vi "GetXML.vi"(0 "Node ROS":T2={"topic port"=0, "Node"="", "topic"="", "type"="", "node port"=0, "error "={"status"=FALSE, "code"=0, "source"=""}, "Direction"=enum."Node", "APIs"=[], "Update (ms)"=1, "write queue"=1}, 1 "Subscribers in":T1(array[cluster])) -> (2 "error IO":errorcluster, 3 "reply":string, 4 "Subscribers Out":T1(array[cluster]))   [LabVIEW 2012]
uses:
  ROSLog.ctl
  _ROSDefinition.vi
  MessageBuilding/std_msgs/subs/i16Scalar.vi
  MessageBuilding/std_msgs/subs/stringScalar.vi
  SubVIs/_ROSDirection.ctl
  SubVIs/_ROSControl.ctl
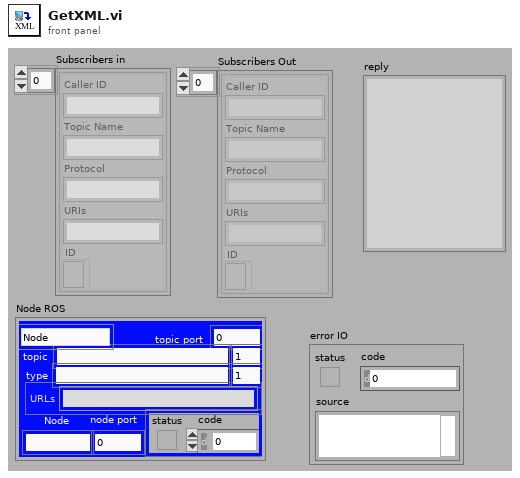
[diagram p1: front panel]
types:
  T1 = cluster{"Caller ID":string, "Topic Name":string, "Protocol":string, "URIs":string, "ID":refnum<k5>}[]
  T2 = typedef "_ROSControl.ctl" = cluster{"topic port":u16, "Node":string, "topic":string, "type":string, "node port":u32, "error ":errorcluster, "Direction":T3, "APIs":string[], "Update (ms)":u16, "write queue":u16}
  T3 = typedef "_ROSDirection.ctl" = enum16{"Node", "Publisher", "Subscriber", "Service Client"}
  T4 = typedef "ROSLog.ctl" = cluster{"Sent":string, "Reply":string, "MethodName":string, "success":bool, "Dir1":string, "Dir2":string, "Time Stamp":string}
  T5 = enum16{"Add Server", "Clear Server", "Clear All", "Get Info", "GetPanelInfo"}
  T6 = cluster{"Caller ID":string, "Topic Name":string, "Protocol":string, "URIs":string, "ID":refnum<k5>}
  T7 = typedef "requestTopic.ctl" = cluster{"New Subscriber":cluster{"Caller ID":string, "Topic Name":string, "Protocol":string, "URIs":string, "ID":refnum<k5>}, "ROS of Server":T2, "new port":u16}
  T8 = typedef "MyState.ctl" = enum16{"No Connection", "Registered", "Connected", "Close"}
  T9 = typedef "ServoInfo.ctl" = cluster{"vi name":string, "VI Refnum":refnum<vi>, "queue":refnum<queue>, "ROS":T2, "notifier":refnum<notifier>}
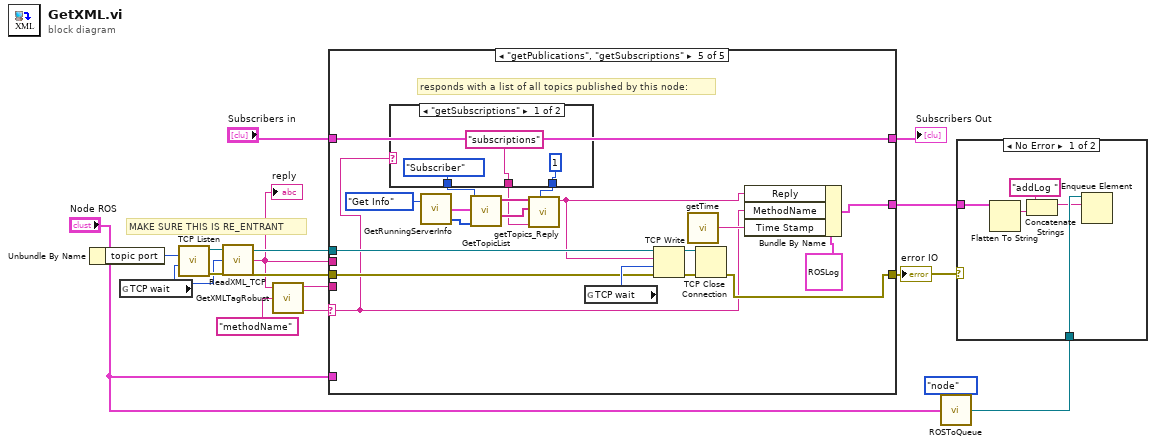
[diagram p0: block diagram]
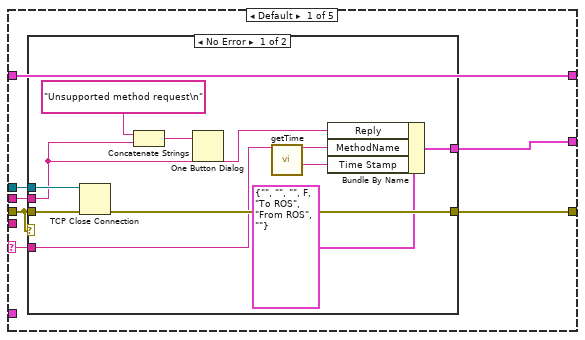
[diagram p3: hidden frame]
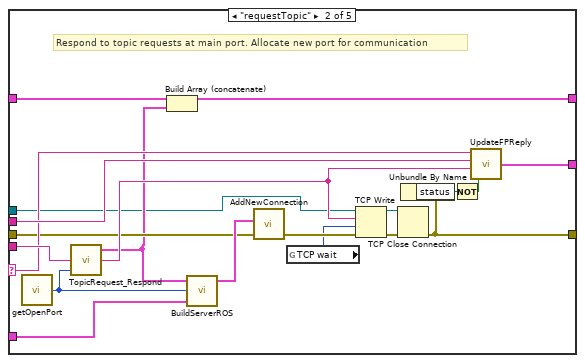
[diagram p5: hidden frame]
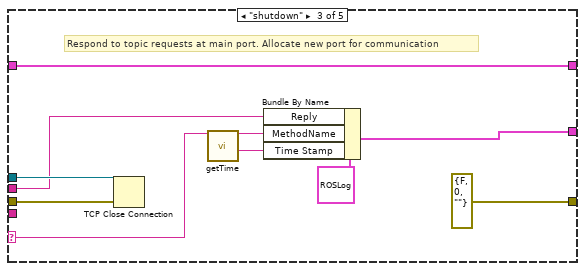
[diagram p6: hidden frame]
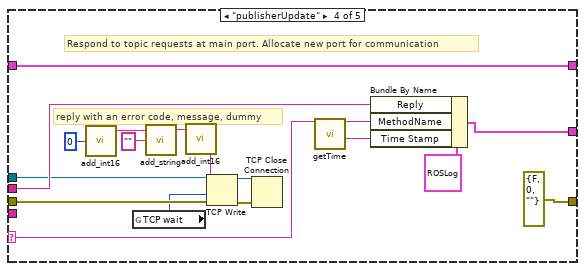
[diagram p7: hidden frame]
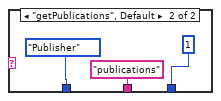
[diagram p8: hidden frame]
diagram:
  # "MAKE SURE THIS IS RE_ENTRANT"
  n1 = Unbundle By Name("Node ROS") -> ("topic port"=w8:u16)
  n2 = global read "_ROSDefinition.vi" "TCP wait"() -> (w1:i32)
  n3 = call <vilib>:"TCP Listen.vi"("timeout ms (wait forever: -1)"=w1, "port"=w8) -> ("error out"=w17:errorcluster, "connection ID"=w16:refnum<k5>)  [unwired: 5 in, 3 out]
  n4 = call "ReadXML_TCP.vi"("error in"=w17, "timeout ms (3000)"=w1, "connection ID in"=w16) -> ("error out"=w14:errorcluster, "data out"=w3:string, "connection ID out"=w13:refnum<k5>)
  "reply" <- w3
  n5 = call "GetXMLTagRobust.vi"("Tag"="methodName", "String"=w3) -> ("value"=w10:string, "String w/o Tag"=w11:string)  [unwired: 1 in, 2 out]
  n6 = case shown="\"getPublications\", \"getSubscriptions\"" w10 {
    selector: w10 -> [w21 w52 w58 w77 w86]
    tunnel: w11 -> [_ w55 _ _ _]
    tunnel: "Subscribers in" -> [w24 w43 w64 w81 w101]
    tunnel: w13 -> [w23 w36 w63 w69 w94]
    tunnel: w14 -> [w19 w45 w62 w70 w93]
    tunnel: [w24 w42 w64 w81 w101] -> w15
    tunnel: "Node ROS" -> [_ w39 _ _ _]
    tunnel: w3 -> [w20 w53 w59 w78 _]
    tunnel: [w22 w46 errorcluster {"status"=FALSE, "code"=0, "source"=""} ("error IO") errorcluster {"status"=FALSE, "code"=0, "source"=""} ("error IO") w87] -> w4
    tunnel: [w18 w41 w56 w75 w100] -> w5
    frame Default {
      n7 = case shown="No Error" w19 {
        tunnel: w23 -> [w34 _]
        tunnel: w19 -> [w33 w35]
        tunnel: [w32 w35] -> w22
        tunnel: [w27 _] -> w18
        tunnel: w21 -> [w26 _]
        tunnel: w20 -> [w25 _]
        frame No Error {
          n8 = TCP Close Connection(connection ID=w34, error in (no error)=w33) -> (error out=w32:errorcluster)  [unwired: 1 in, 1 out]
          n9 = Concatenate Strings("Unsupported method request\n" ("message"), w25) -> (w30:string)
          n10 = One Button Dialog(message=w30) -> ()  [unwired: 1 in, 1 out]
          n11 = call "getTime.vi"() -> ("Current Time"=w28:string)  [unwired: 1 in]
          n12 = Bundle By Name(cluster=T4 {"Sent"="", "Reply"="", "MethodName"="", "success"=FALSE, "Dir1"="To ROS", "Dir2"="From ROS", "Time Stamp"=""} ("Log"), "Reply"=w25, "MethodName"=w26, "Time Stamp"=w28) -> (w27:T4)
        }
        frame Error {
        }
      }
    }
    frame "requestTopic" {
      # "Respond to topic requests at main port. Allocate new port for communication"
      n13 = call "getOpenPort.vi"() -> ("port"=w38:u16)
      n14 = call "TopicRequest_Respond.vi"("port"=w38, "XML"=w55) -> ("Topic Request Reply"=w51:string, "New Subscriber"=w37:T6)  [unwired: 2 in]
      n15 = Build Array (concatenate)(w43, w37) -> (w42:T1)
      n16 = call "BuildServerROS.vi"("Node ROS"=w39, "port"=w38, "New Subscriber"=w37) -> ("data"=w47:T7)  [unwired: 2 in]
      n17 = call "AddNewConnection.vi"("error in (no error)"=w45, "data"=w47) -> ("error out"=w44:errorcluster)  [unwired: 3 in]
      n18 = global read "_ROSDefinition.vi" "TCP wait"() -> (w40:i32)
      n19 = TCP Write(connection ID=w36, data in=w51, error in (no error)=w44, 9:w40) -> (connection ID out=w54:refnum<k5>, error out=w48:errorcluster)  [unwired: 1 out]
      n20 = TCP Close Connection(connection ID=w54, error in (no error)=w48) -> (error out=w46:errorcluster)  [unwired: 1 in, 1 out]
      n21 = Unbundle By Name(w46) -> ("status"=w50:bool)
      n22 = Not(x=w50) -> (.not. x?=w49:bool)
      n23 = call "UpdateFPReply.vi"("success?"=w49, "Reply"=w51, "Sent"=w53, "method"=w52) -> ("Log"=w41:T4)
    }
    frame "shutdown" {
      # "Respond to topic requests at main port. Allocate new port for communication"
      n24 = TCP Close Connection(connection ID=w63, error in (no error)=w62) -> ()  [unwired: 1 in, 2 out]
      n25 = call "getTime.vi"() -> ("Current Time"=w57:string)  [unwired: 1 in]
      n26 = Bundle By Name(cluster=T4 {"Sent"="", "Reply"="", "MethodName"="", "success"=FALSE, "Dir1"="To ROS", "Dir2"="From ROS", "Time Stamp"=""} ("Log"), "Reply"=w59, "MethodName"=w58, "Time Stamp"=w57) -> (w56:T4)
    }
    frame "publisherUpdate" {
      # "reply with an error code, message, dummy"
      # "Respond to topic requests at main port. Allocate new port for communication"
      n27 = call-poly "add_int16.vi"("Numeric"=i16 0) -> ("msg out"=w74:string)  [unwired: 4 in]
      n28 = global read "_ROSDefinition.vi" "TCP wait"() -> (w68:i32)
      n29 = call-poly "add_string.vi"("String"="", "msg in"=w74) -> ("msg out"=w73:string)  [unwired: 3 in]
      n30 = call-poly "add_int16.vi"("msg in"=w73) -> ("msg out"=w67:string)  [unwired: 4 in]
      n31 = TCP Write(connection ID=w69, data in=w67, error in (no error)=w70, 9:w68) -> (connection ID out=w66:refnum<k5>, error out=w65:errorcluster)  [unwired: 1 out]
      n32 = TCP Close Connection(connection ID=w66, error in (no error)=w65) -> ()  [unwired: 1 in, 2 out]
      n33 = call "getTime.vi"() -> ("Current Time"=w76:string)  [unwired: 1 in]
      n34 = Bundle By Name(cluster=T4 {"Sent"="", "Reply"="", "MethodName"="", "success"=FALSE, "Dir1"="To ROS", "Dir2"="From ROS", "Time Stamp"=""} ("Log"), "Reply"=w78, "MethodName"=w77, "Time Stamp"=w76) -> (w75:T4)
    }
    frame "getPublications", "getSubscriptions" {
      # "responds with a list of all topics published by this node:"
      n35 = case shown="\"getSubscriptions\"" w86 {
        tunnel: [_ROSDirection."Subscriber" ("ROS.Direction") _ROSDirection."Publisher" ("ROS.Direction")] -> w85
        tunnel: [1 ("Code") 1 ("Code")] -> w83
        tunnel: ["subscriptions" ("StatusMessage") "publications" ("StatusMessage")] -> w82
        frame "getSubscriptions" {
        }
        frame "getPublications", Default {
        }
      }
      n36 = call "GetRunningServerInfo.vi"("Task"=T5."Get Info") -> ("Status"=w90:T8[], "servers"=w91:T9[])  [unwired: 1 in, 1 out]
      n37 = call "GetTopicList.vi"("Status"=w90, "servers"=w91, "ROS.Direction"=w85) -> ("Topic Types"=w84:string[], "Topics"=w89:string[])  [unwired: 7 in]
      n38 = call "getTopics_Reply.vi"("Code"=w83, "StatusMessage"=w82, "Topic Types"=w84, "Topics"=w89) -> ("XML Out"=w88:string)  [unwired: 7 in]
      n39 = global read "_ROSDefinition.vi" "TCP wait"() -> (w97:i32)
      n40 = TCP Write(connection ID=w94, data in=w88, error in (no error)=w93, 9:w97) -> (connection ID out=w95:refnum<k5>, error out=w96:errorcluster)  [unwired: 1 out]
      n41 = call "getTime.vi"() -> ("Current Time"=w98:string)  [unwired: 1 in]
      n42 = TCP Close Connection(connection ID=w95, error in (no error)=w96) -> (error out=w87:errorcluster)  [unwired: 1 in, 1 out]
      n43 = Bundle By Name(cluster=T4 {"Sent"="", "Reply"="", "MethodName"="", "success"=FALSE, "Dir1"="To ROS", "Dir2"="From ROS", "Time Stamp"=""} ("Log"), "Reply"=w88, "MethodName"=w86, "Time Stamp"=w98) -> (w100:T4)
    }
  }
  "error IO" <- w4
  "Subscribers Out" <- w15
  n44 = call "ROSToQueue.vi"("ROS"="Node ROS", "Name"=enum16{"topic", "node"}."node") -> ("queue"=w6:refnum<queue>)  [unwired: 2 in, 1 out]
  n45 = case shown="No Error" w4 {
    tunnel: w6 -> [w112 _]
    tunnel: w5 -> [w111 _]
    frame No Error {
      n46 = Flatten To String(anything=w111) -> (data string=w109:string)  [unwired: 3 in, 2 out]
      n47 = Concatenate Strings("addLog " ("string"), w109) -> (w110:string)
      n48 = Enqueue Element(queue=w112, element=w110) -> ()  [unwired: 2 in, 3 out]
    }
    frame Error {
    }
  }
